vi "LinearBearingControl.vi"() -> ()   [LabVIEW 2012]
uses:
  stressTestTypeDef.ctl
  <vilib>/Utility/error.llb/DialogType.ctl
  allStatesTypeDef.ctl
  <vilib>/Analysis/baseanly.llb/Mean (DBL).vi
  <vilib>/Utility/file.llb/Write To Spreadsheet File (DBL).vi
  <resource>/objmgr/daqmx.rc
  <vilib>/Analysis/NI_AALBase.lvlib
panel:
  out "Force":dbl[](array[numeric]) format="%#.2g"
  out "Measurement":dbl[](graph)
  out "Bias (N)":dbl
  in  "Channel Parameters":T1={"Maximum Value"=10.0, "Minimum Value"=-10.0, "Channel"="Dev2/ai7"}
  in  "pulse/rev":u16(ring)=25600 items=["400"=400, "800"=800, "1600"=1600, "3200"=3200, "6400"=6400, "12800"=12800, "25600"=25600]
  out "concatenated string":string
  out "rigid body LED":bool
  out "strain rate":dbl
  in  "chain L0":i32=230
  out "mm/s (timed)":dbl
  in  "Direction":bool
  in  "Only Move Lin":bool
  out "writing data":bool
  out "stop sys":bool
  out "udp error out":errorcluster
  out "Voltages":dbl[](array[numeric])
  in  "Start System":bool
  in  "Auto Bias":bool=TRUE
  in  "Unbias":bool
  in  "Bias":bool
  in  "Collect Data":bool=TRUE
  in  "Timing parameters":T2={"Sample Rate"=1000.0, "Samples to Read"=100}
  out "filenameOut":string
  in  "Optitrack Parameters":T3={"Optitrack IP"="130.207.141.229", "Optitrack Port"=1520, "timeout (sec)"=80}
  out "Data Output File":path
  in  "Output Folder":path=path "C:/Users/Administrator/Dropbox/expData/chainData"
  in  "Program Parameters":T5={"v"=2500, "Iters"=2, "Speed"=5, "Delay"=0.5, "H"=11.5, "SD"=10, "Name"="Stretch", "Type"=enum."FRACT ON"} {"Speed" min=0 max=49 step=5}
  out "strain %":dbl
  out "FT error out":errorcluster
  # "for 6 smarts\nSDmax ~ 170mm"
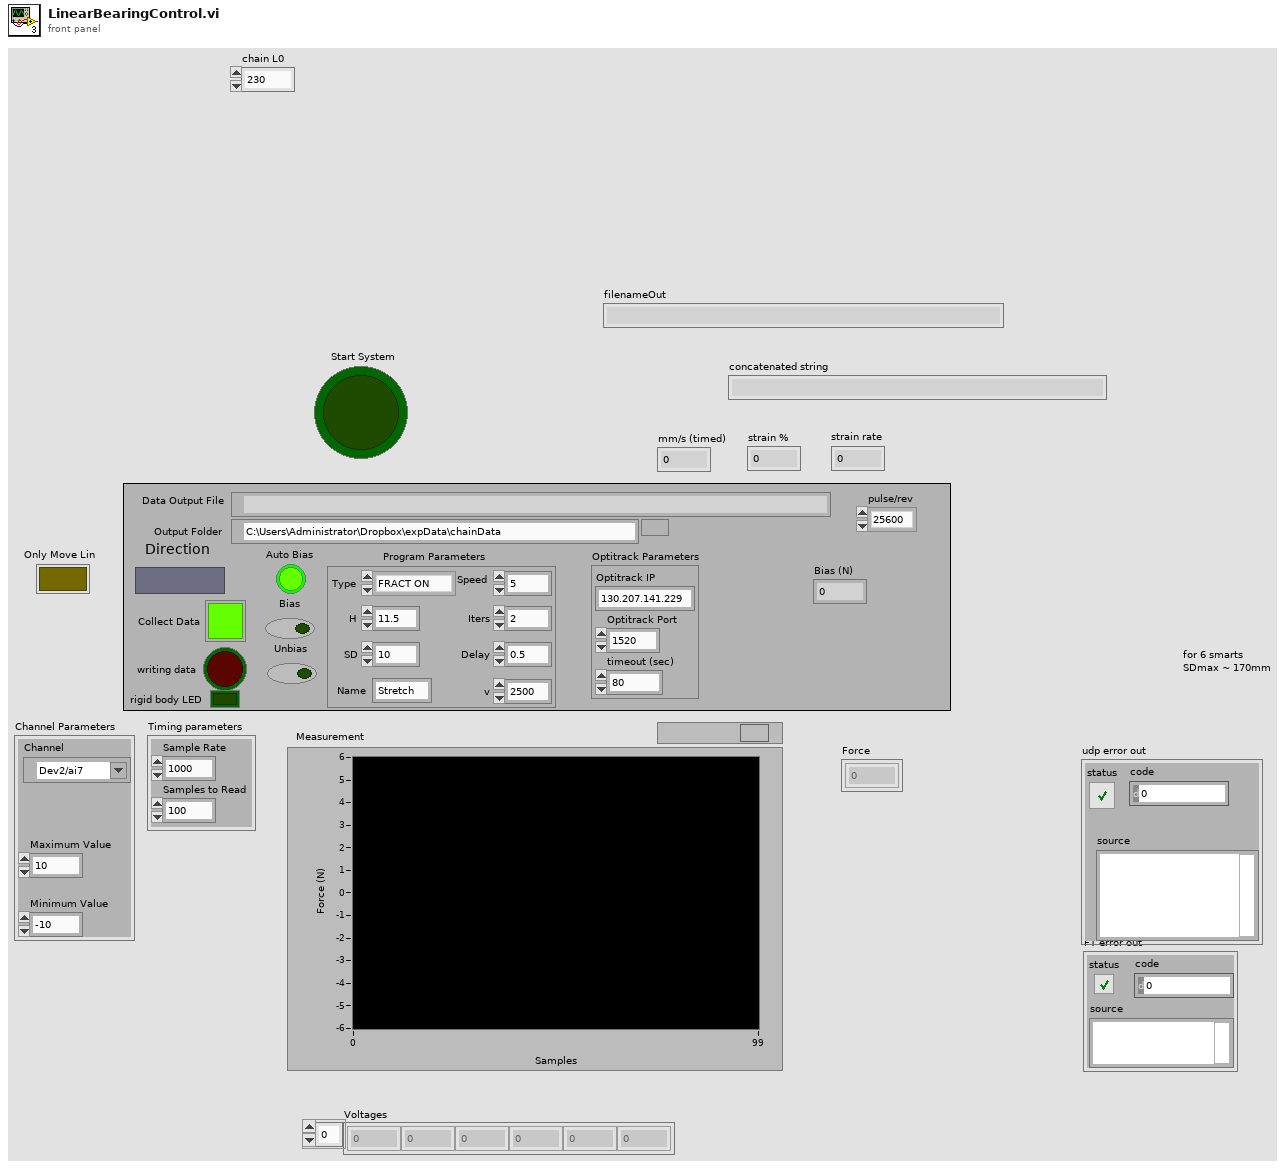
[diagram p1: front panel]
types:
  T1 = cluster{"Maximum Value":dbl, "Minimum Value":dbl, "Channel":tag}
  T2 = cluster{"Sample Rate":dbl, "Samples to Read":i32}
  T3 = cluster{"Optitrack IP":string, "Optitrack Port":u16, "timeout (sec)":i32}
  T4 = typedef "stressTestTypeDef.ctl" = enum16{"OFF", "ON", "EXTEND", "SPRING", "FRACT ON", "SAC", "FRACT SAC"}
  T5 = cluster{"v":i32, "Iters":i32, "Speed":i32, "Delay":dbl, "H":dbl, "SD":i32, "Name":string, "Type":T4}
  T6 = cluster{"distance mm":i32, "Direction":bool, "device name":tag, "speed (mm/s)":i32, "pulse/rev":u16}
  T7 = typedef "DialogType.ctl" = u16
  T8 = cluster{"SD":i32, "Delay":dbl, "Speed":i32, "Iters":i32, "Type":T4, "timeout":i32}
  T9 = typedef "allStatesTypeDef.ctl" = enum16{"open udp", "start record", "recording", "move linear actuator", "end record", "close udp", "end"}
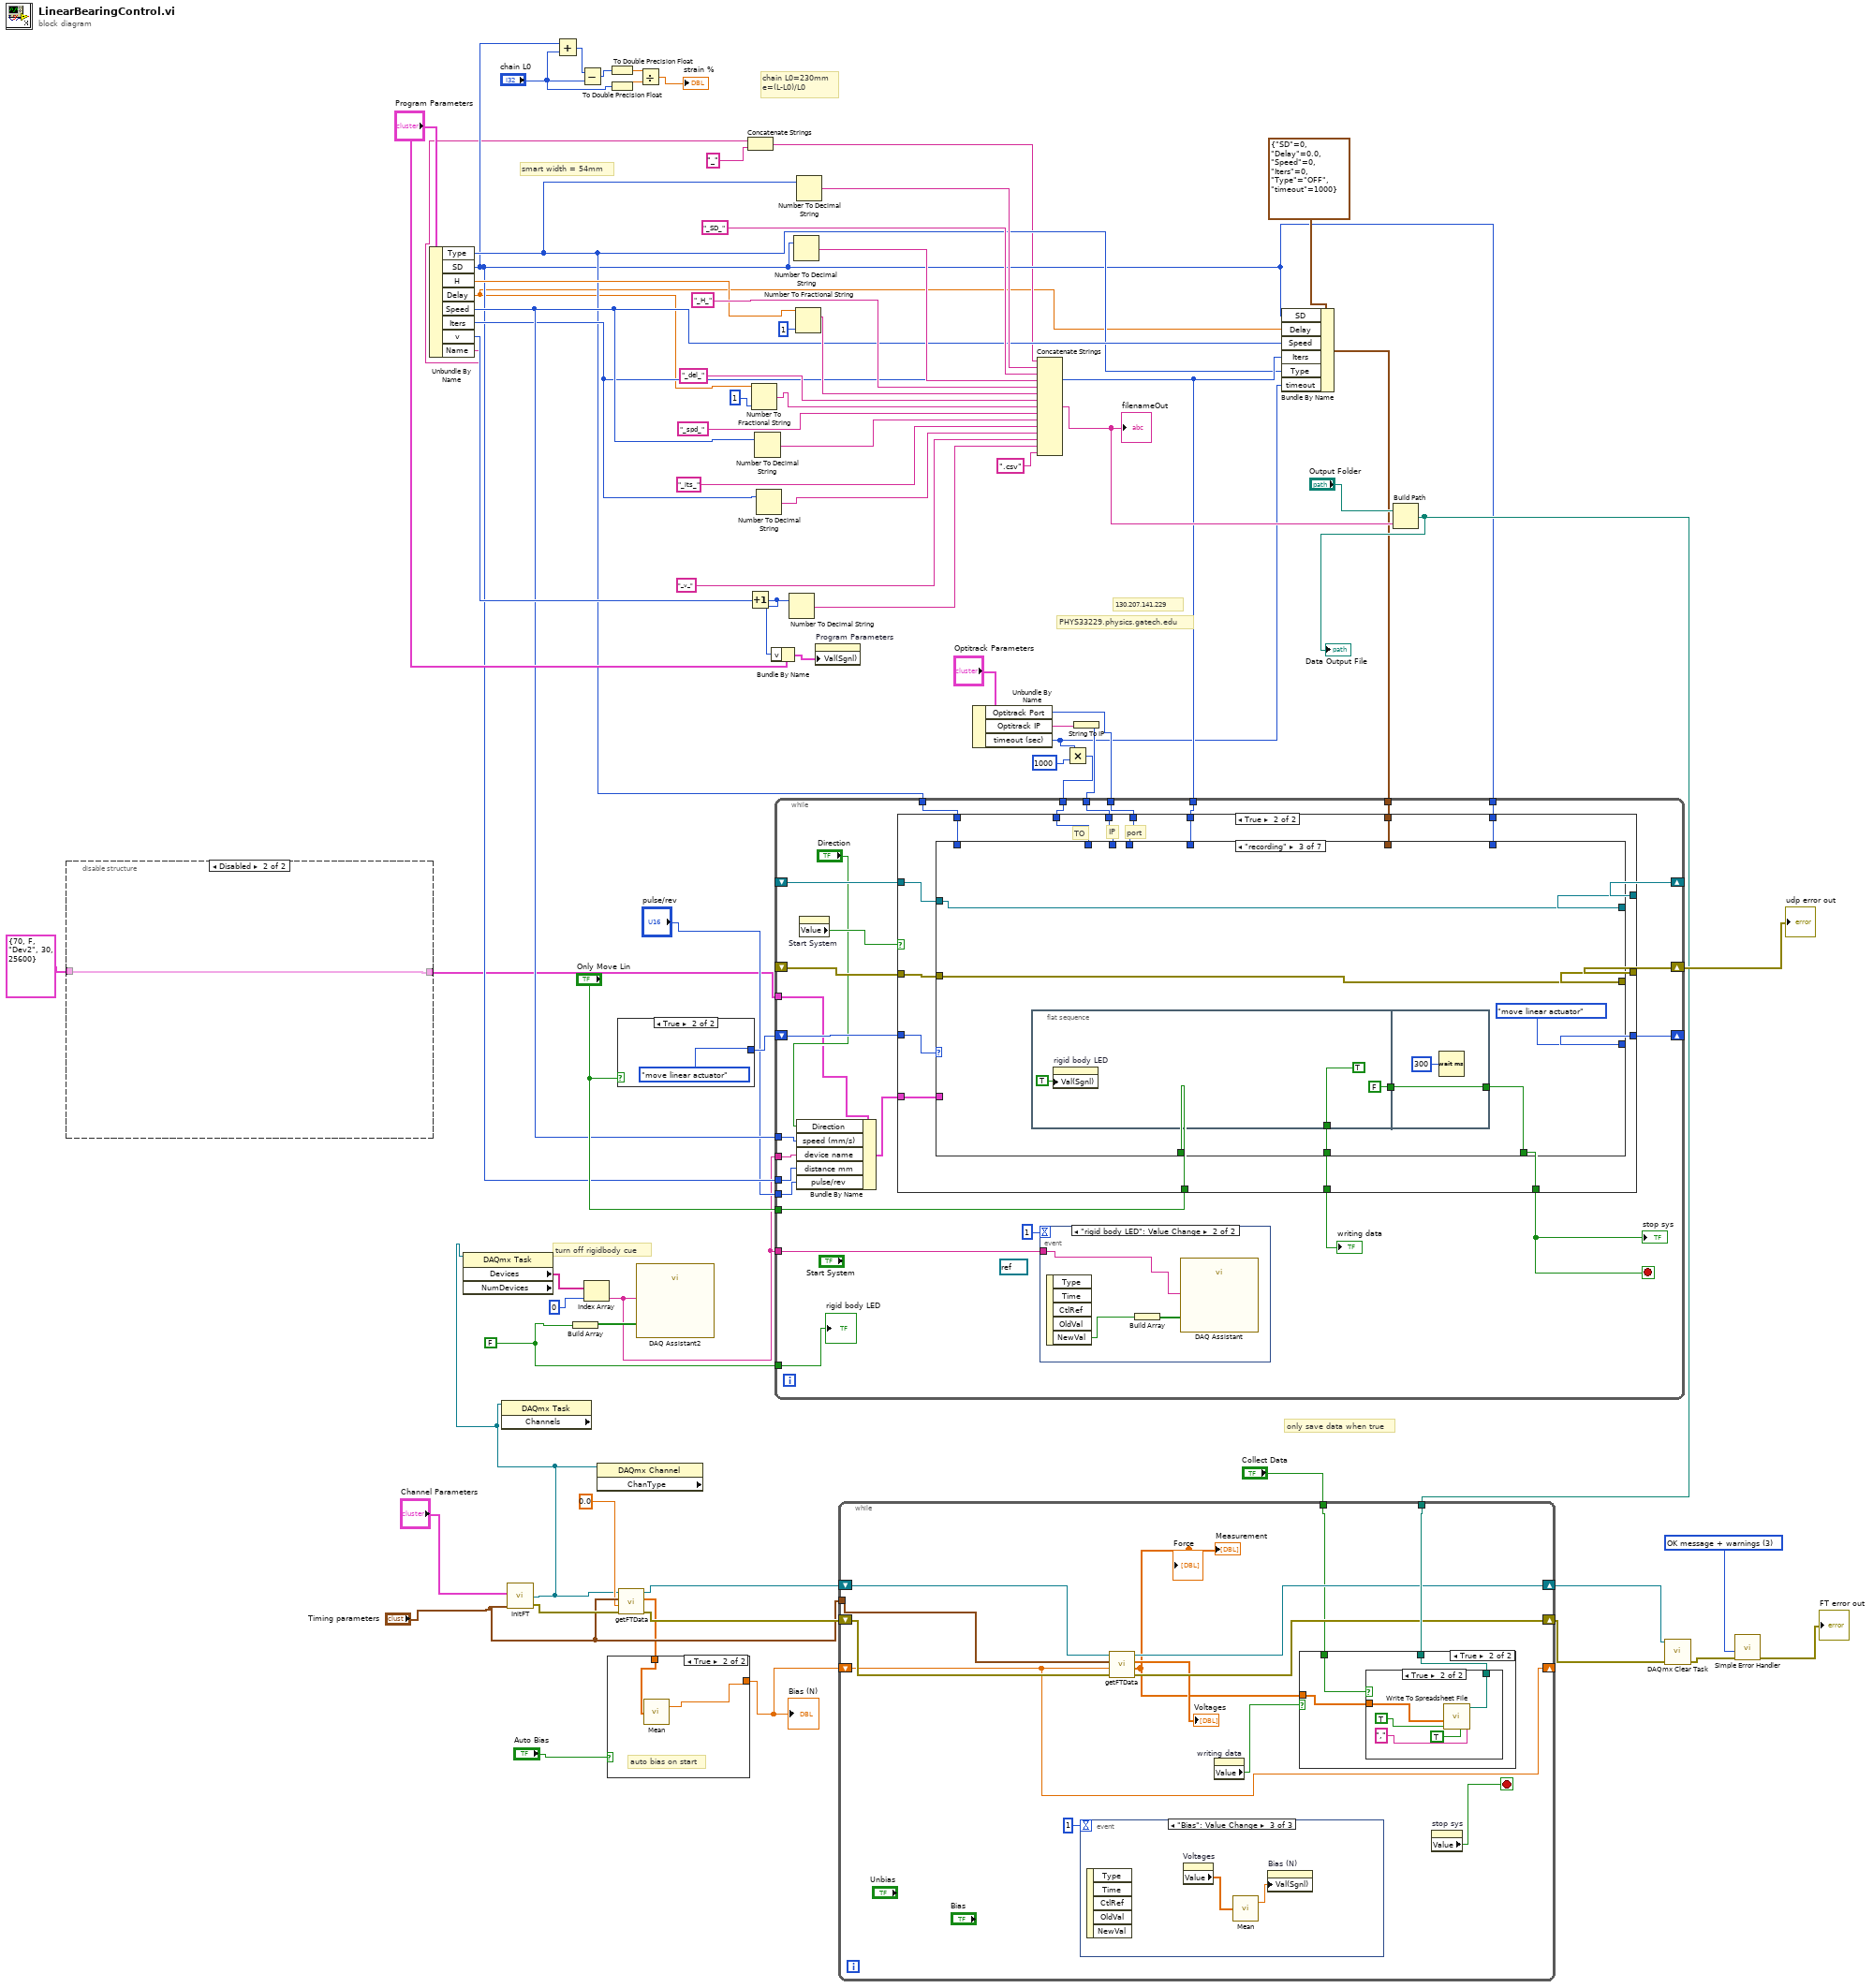
[diagram p0: block diagram]
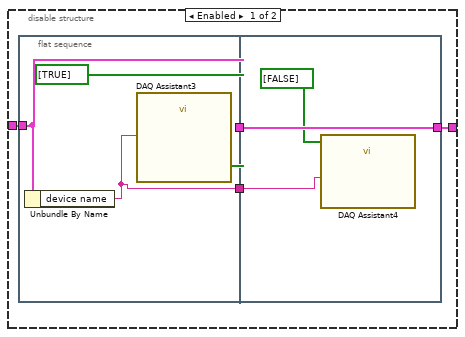
[diagram p2: hidden frame]
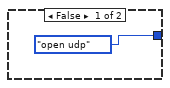
[diagram p3: hidden frame]
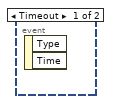
[diagram p4: hidden frame]
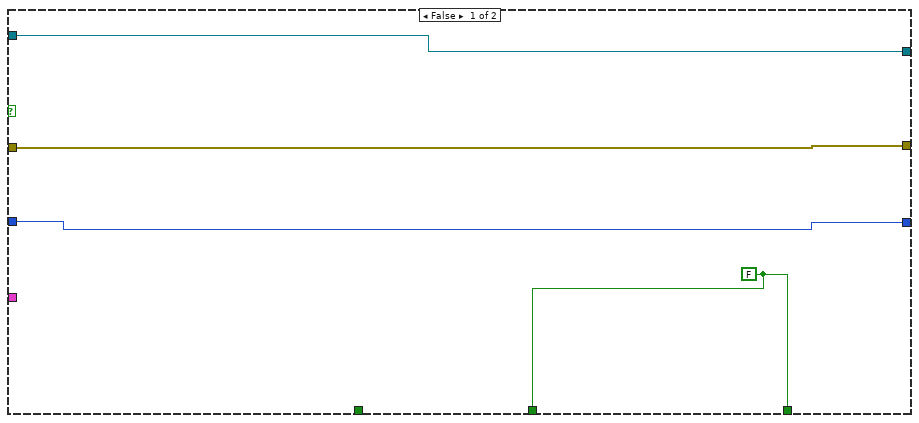
[diagram p5: hidden frame]
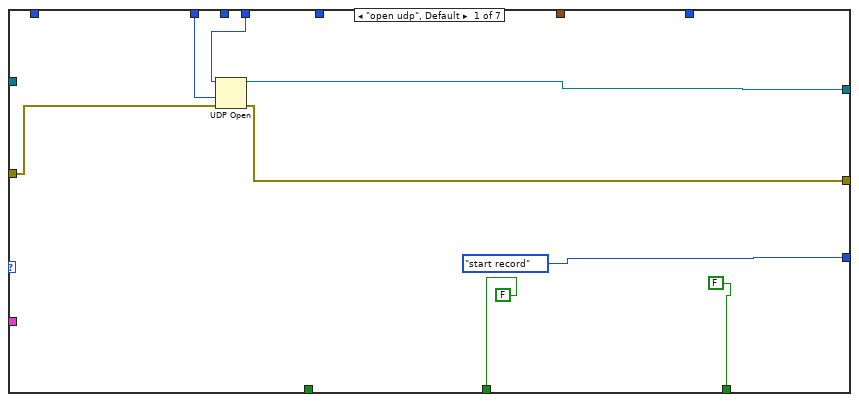
[diagram p6: hidden frame]
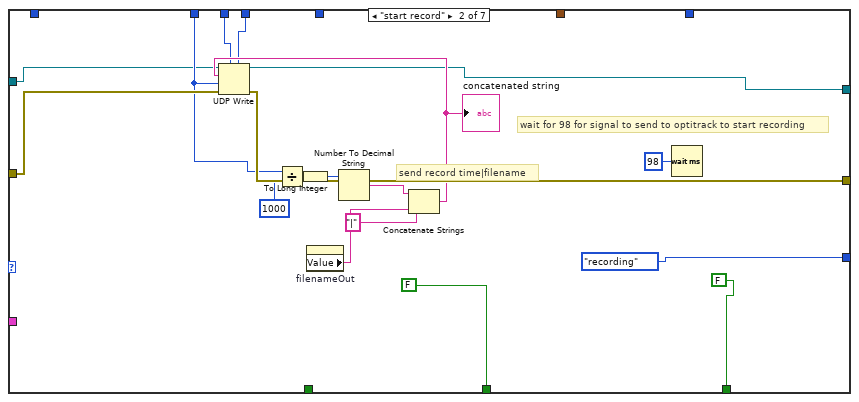
[diagram p7: hidden frame]
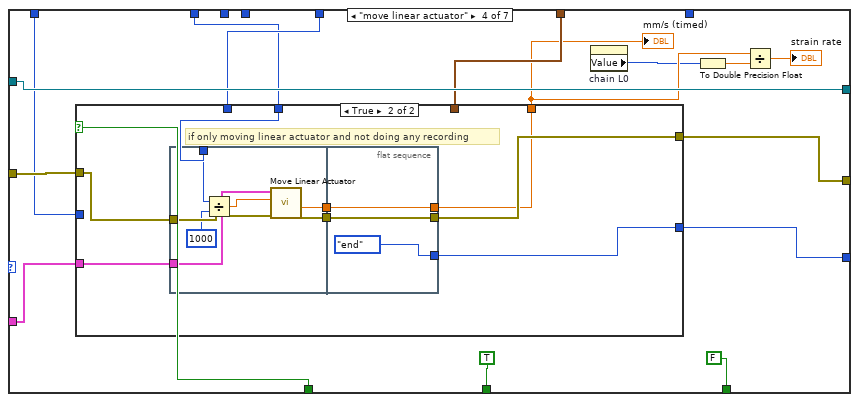
[diagram p8: hidden frame]
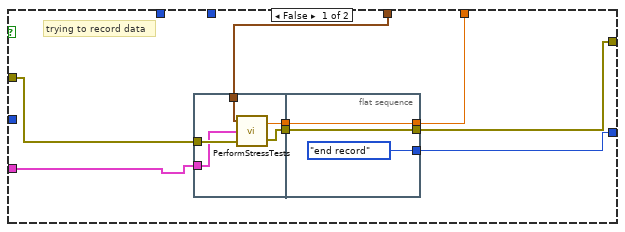
[diagram p9: hidden frame]
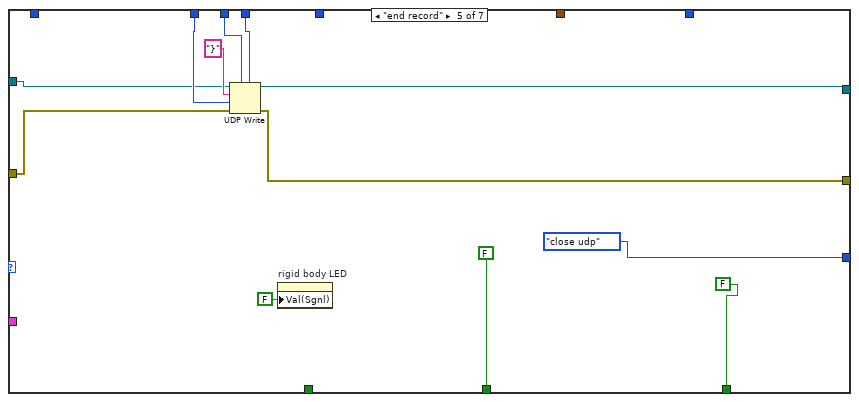
[diagram p10: hidden frame]
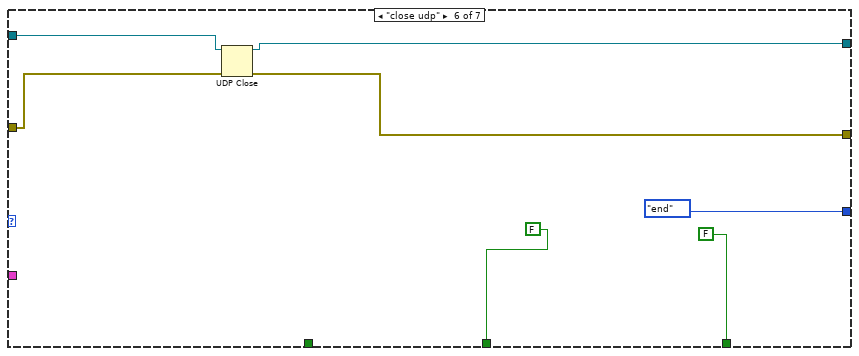
[diagram p11: hidden frame]
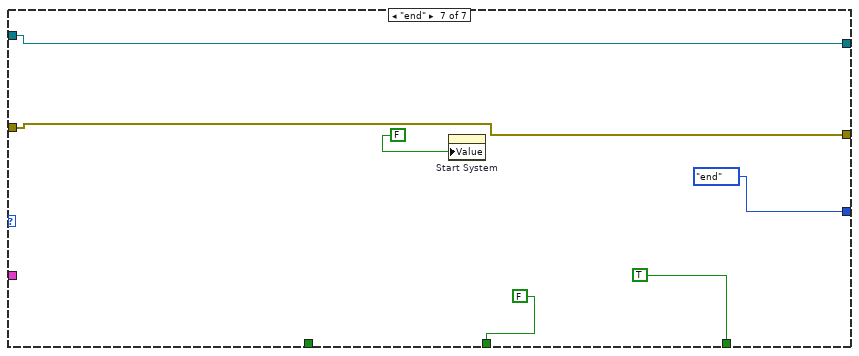
[diagram p12: hidden frame]
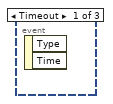
[diagram p13: hidden frame]
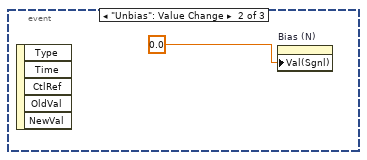
[diagram p14: hidden frame]
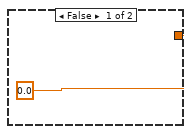
[diagram p17: hidden frame]
diagram:
  w19 = FALSE
  w47 = T7 3 items=["no dialog", "OK message", "continue or stop message", "OK message + warnings", "continue/stop + warnings"] ("type of dialog (OK msg:1)")
  # "turn off rigidbody cue"
  # "chain L0=230mm\ne=(L-L0)/L0"
  # "only save data when true"
  # "smart width = 54mm"
  # "PHYS33229.physics.gatech.edu"
  # "130.207.141.229"
  n1 = disable-structure shown="Disabled" {
    disable-tunnel: [w76 w85] -> w10
    disable-tunnel: T6 {"distance mm"=70, "Direction"=FALSE, "device name"="Dev2", "speed (mm/s)"=30, "pulse/rev"=25600} ("linear actuator info") -> [w75 w85]
    frame Enabled {
      n2 = flat-sequence {
        tunnel: w75 -> [w81]
        tunnel: [w81] -> w78
        tunnel: [w79] -> w77
        tunnel: [w84] -> w76
        tunnel: w78 -> [w84]
        tunnel: w77 -> [w83]
        frame #0 {
          n3 = Unbundle By Name(w81) -> ("device name"=w79:tag)
          n4 = call "DAQ Assistant3"("data"=bool[] [TRUE], "device name"=w79) -> ()  [unwired: 16 in, 2 out]
        }
        frame #1 {
          n5 = call "DAQ Assistant4"("data"=bool[] [FALSE], "device name"=w83) -> ()  [unwired: 16 in, 2 out]
        }
      }
    }
    frame Disabled {
    }
  }
  n6 = Unbundle By Name("Program Parameters") -> ("Type"=w29:T4, "SD"=w21:i32, "H"=w56:dbl, "Delay"=w13:dbl, "Speed"=w31:i32, "Iters"=w30:i32, "v"=w57:i32, "Name"=w16:string)
  n7 = call "InitFT.vi"("Timing parameters"="Timing parameters", "Channel Parameters"="Channel Parameters") -> ("error out"=w44:errorcluster, "task out"=w6:refnum<k21>)  [unwired: 3 in]
  n8 = property class="DAQmx Task" props=["Devices", "NumDevices"](reference=w6) -> ("Devices"=w3:tag[])  [unwired: 1 in, 3 out]
  n9 = property class="DAQmx Task" props=["Channels"](reference=w6) -> ()  [unwired: 1 in, 3 out]
  n10 = Add(x=w21, y="chain L0") -> (x+y=w27:i32)
  n11 = Build Array(w19) -> (w20:bool[])
  n12 = Subtract(x=w27, y="chain L0") -> (x-y=w26:i32)
  n13 = Index Array(array=w3, index=0) -> (element=w5:tag)
  n14 = property class="DAQmx Channel" props=["ChanType"](reference=w6) -> ()  [unwired: 1 in, 3 out]
  n15 = To Double Precision Float(number=w26) -> (double precision float=w24:dbl)
  n16 = To Double Precision Float(number="chain L0") -> (double precision float=w23:dbl)
  n17 = case shown="True" "Only Move Lin" {
    tunnel: [allStatesTypeDef."open udp" allStatesTypeDef."move linear actuator"] -> w74
    frame False {
    }
    frame True {
    }
  }
  n18 = call "getFTData.vi"("error in"=w44, "bias"=0.0, "Timing parameters"="Timing parameters", "task in"=w6) -> ("error out"=w40:errorcluster, "Voltage"=w2:dbl[], "task out 2"=w41:refnum<k21>)  [unwired: 1 in, 1 out]
  n19 = case shown="True" "Auto Bias" {
    tunnel: w2 -> [_ w90]
    tunnel: [0.0 ("Bias (N) 2") w89] -> w1
    frame False {
    }
    frame True {
      # "auto bias on start"
      n20 = call-poly <vilib>:"Mean.vi"("X"=w90) -> ("mean"=w89:dbl)  [unwired: 1 out]
    }
  }
  "Bias (N)" <- w1
  n21 = call "DAQ Assistant2"("data"=w20, "device name"=w5) -> ()  [unwired: 16 in, 2 out]
  n22 = Divide(x=w24, y=w23) -> (x/y=→"strain %":dbl)
  n23 = Concatenate Strings(w16, "_") -> (w17:string)
  n24 = Increment(x=w57) -> (x+1=w58:i32)
  n25 = Number To Fractional String(number=w13, precision (6)=i16 1) -> (F-format string=w11:string)  [unwired: 2 in]
  n26 = Number To Decimal String(number=w31) -> (decimal integer string=w62:string)  [unwired: 1 in]
  n27 = Number To Decimal String(number=w30) -> (decimal integer string=w60:string)  [unwired: 1 in]
  n28 = Bundle By Name(cluster="Program Parameters", "v"=w58) -> (w54:T5)
  n29 = Number To Decimal String(number=w58) -> (decimal integer string=w64:string)  [unwired: 1 in]
  n30 = Number To Decimal String(number=w21) -> (decimal integer string=w70:string)  [unwired: 1 in]
  n31 = Number To Fractional String(number=w56, precision (6)=i16 1) -> (F-format string=w67:string)  [unwired: 2 in]
  n32 = Number To Decimal String(number=w29) -> (decimal integer string=w72:string)  [unwired: 1 in]
  n33 = property on="Program Parameters" class="Clust (strict)"("Val(Sgnl)"=w54) -> ()  [unwired: 2 in, 2 out]
  n34 = Unbundle By Name("Optitrack Parameters") -> ("Optitrack Port"=w52:u16, "Optitrack IP"=w51:string, "timeout (sec)"=w15:i32)
  n35 = Concatenate Strings(w17, w72, "_SD_", w70, "_H_", w67, "_del_", w11, "_spd_", w62, "_its_", w60, "_v_", w64, ".csv") -> (w33:string)
  "filenameOut" <- w33
  n36 = Multiply(x=w15, y=1000) -> (x*y=w48:i32)
  n37 = String To IP(1:w51) -> (0:w50:u32)
  n38 = Bundle By Name(cluster=T8 {"SD"=0, "Delay"=0.0, "Speed"=0, "Iters"=0, "Type"=enum."OFF", "timeout"=1000}, "SD"=w21, "Delay"=w13, "Speed"=w31, "Iters"=w30, "Type"=w29, "timeout"=w15) -> (w28:T8)
  n39 = while {
    shift-right: [w117] -> w36
    shift-left: _ -> [w116]
    shift-right: [w114] -> _
    shift-left: w74 -> [w115]
    tunnel: w52 -> [w112]
    tunnel: w50 -> [w113]
    tunnel: w48 -> [w93]
    shift-right: [w111] -> _
    shift-left: _ -> [w110]
    tunnel: "Only Move Lin" -> [w107]
    tunnel: w31 -> [w104]
    tunnel: w21 -> [w95]
    tunnel: w29 -> [w103]
    tunnel: w30 -> [w102]
    tunnel: w28 -> [w101]
    tunnel: w21 -> [w99]
    tunnel: w19 -> [w98]
    tunnel: w5 -> [w96]
    tunnel: w5 -> [w94]
    tunnel: "pulse/rev" -> [w92]
    tunnel: w10 -> [w91]
    stop <- w109 stop-if-true
    (unwired) refnum<k21> refnum ("Name")
    n40 = Bundle By Name(cluster=w91, "Direction"="Direction", "speed (mm/s)"=w104, "device name"=w96, "distance mm"=w95, "pulse/rev"=w92) -> (w106:T6)
    n41 = property on="Start System" class="Bool (strict)"() -> ("Value"=w108:bool)  [unwired: 2 in, 2 out]
    n42 = case shown="True" w108 {
      tunnel: [w121 w141] -> w117
      tunnel: w116 -> [w121 w140]
      tunnel: w115 -> [w124 w139]
      tunnel: [w124 w138] -> w114
      tunnel: w113 -> [_ w137]
      tunnel: w112 -> [_ w130]
      tunnel: w93 -> [_ w136]
      tunnel: [w122 w135] -> w111
      tunnel: w110 -> [w122 w134]
      tunnel: [w123 w133] -> w100
      tunnel: [w123 w132] -> w109
      tunnel: w107 -> [_ w131]
      tunnel: w106 -> [_ w129]
      tunnel: w103 -> [_ w128]
      tunnel: w102 -> [_ w127]
      tunnel: w101 -> [_ w126]
      tunnel: w99 -> [_ w125]
      frame False {
        w123 = FALSE
      }
      frame True {
        # "IP"
        # "TO"
        # "port"
        n43 = case shown="\"recording\"" w139 {
          tunnel: w136 -> [w146 w159 _ w179 w236 _ _]
          tunnel: w140 -> [w147 w165 w169 w190 w240 w246 w248]
          tunnel: [w148 w166 w169 w189 w239 w247 w248] -> w141
          tunnel: [allStatesTypeDef."start record" allStatesTypeDef."recording" allStatesTypeDef."move linear actuator" w192 allStatesTypeDef."close udp" allStatesTypeDef."end" allStatesTypeDef."end"] -> w138
          tunnel: [FALSE FALSE w171 FALSE FALSE FALSE TRUE] -> w132
          tunnel: w137 -> [_ w152 _ _ w230 _ _]
          tunnel: [w145 w155 w170 w191 w234 w245 w253] -> w135
          tunnel: w134 -> [_ w156 w170 w191 w233 w241 w253]
          tunnel: [FALSE FALSE w172 TRUE FALSE FALSE FALSE] -> w133
          tunnel: w131 -> [_ _ _ w188 _ _ _]
          tunnel: w130 -> [w142 w151 _ _ w231 _ _]
          tunnel: w129 -> [_ _ _ w187 _ _ _]
          tunnel: w128 -> [_ _ _ w185 _ _ _]
          tunnel: w127 -> [_ _ _ w186 _ _ _]
          tunnel: w126 -> [_ _ _ w184 _ _ _]
          tunnel: w125 -> [_ _ _ _ _ _ _]
          frame "open udp", Default {
            n44 = UDP Open(8:w147, 9:w146, 11:w142) -> (port=w145:refnum<k16>, 0:w148:errorcluster)  [unwired: 2 in, 1 out]
          }
          frame "start record" {
            # "wait for 98 for signal to send to optitrack to start recording"
            # "send record time|filename"
            n45 = Divide(x=w159, y=1000) -> (x/y=w158:dbl)
            n46 = To Long Integer(number=w158) -> (32bit integer=w157:i32)
            n47 = property on="filenameOut" class="Str"() -> ("Value"=w163:string)  [unwired: 2 in, 2 out]
            n48 = Number To Decimal String(number=w157) -> (decimal integer string=w161:string)  [unwired: 1 in]
            n49 = Concatenate Strings(w161, "|" ("string"), w163) -> (w162:string)
            "concatenated string" <- w162
            n50 = UDP Write(address=w152, port or service name=w151, connection ID=w156, data in=w162, 8:w165, 9:w159) -> (error out=w166:errorcluster, 3:w155:refnum<k16>)
            n51 = Wait (ms)(milliseconds to wait=u32 98) -> ()  [unwired: 1 out]
          }
          frame "recording" {
            n52 = flat-sequence {
              tunnel: [TRUE] -> w172
              tunnel: [FALSE] -> w168
              tunnel: [w178] -> w171
              tunnel: w168 -> [w178]
              frame #0 {
                n53 = property on="rigid body LED" class="Bool (strict)"("Val(Sgnl)"=TRUE ("Value (Signaling)")) -> ()  [unwired: 2 in, 2 out]
              }
              frame #1 {
                n54 = Wait (ms)(milliseconds to wait=u32 300) -> ()  [unwired: 1 out]
              }
            }
          }
          frame "move linear actuator" {
            n55 = case shown="True" w188 {
              tunnel: [w195 w212] -> w192
              tunnel: w190 -> [w199 w216]
              tunnel: [w198 w217] -> w189
              tunnel: w187 -> [w200 w218]
              tunnel: [w201 w215] -> w183
              tunnel: w186 -> [_ _]
              tunnel: w185 -> [_ _]
              tunnel: w184 -> [w202 _]
              tunnel: w179 -> [_ w211]
              frame False {
                # "trying to record data"
                n56 = flat-sequence {
                  tunnel: w202 -> [w207]
                  tunnel: w200 -> [w203]
                  tunnel: w199 -> [w205]
                  tunnel: [w206] -> w197
                  tunnel: [w204] -> w196
                  tunnel: w197 -> [w210]
                  tunnel: w196 -> [w209]
                  tunnel: [w210] -> w201
                  tunnel: [w209] -> w198
                  tunnel: [allStatesTypeDef."end record"] -> w195
                  frame #0 {
                    n57 = call "PerformStressTests.vi"("error in"=w205, "linear actuator info"=w203, "Test Info"=w207) -> ("error out"=w204:errorcluster, "mm/s (timed)"=w206:dbl)
                  }
                  frame #1 {
                  }
                }
              }
              frame True {
                # "if only moving linear actuator and not doing any recording"
                n58 = flat-sequence {
                  tunnel: w218 -> [w225]
                  tunnel: w216 -> [w223]
                  tunnel: [w224] -> w214
                  tunnel: [w222] -> w213
                  tunnel: w211 -> [w220]
                  tunnel: w214 -> [w228]
                  tunnel: w213 -> [w227]
                  tunnel: [w228] -> w217
                  tunnel: [w227] -> w215
                  tunnel: [allStatesTypeDef."end"] -> w212
                  frame #0 {
                    n59 = Divide(x=w220, y=1000) -> (x/y=w219:dbl)
                    n60 = call "Move Linear Actuator.vi"("error in"=w223, "timeout"=w219, "linear actuator info"=w225) -> ("error out"=w224:errorcluster, "mm/s (timed)"=w222:dbl)  [unwired: 1 in, 1 out]
                  }
                  frame #1 {
                  }
                }
              }
            }
            "mm/s (timed)" <- w183
            n61 = property on="chain L0" class="DigNum (strict)"() -> ("Value"=w182:i32)  [unwired: 2 in, 2 out]
            n62 = To Double Precision Float(number=w182) -> (double precision float=w181:dbl)
            n63 = Divide(x=w183, y=w181) -> (x/y=→"strain rate":dbl)
          }
          frame "end record" {
            n64 = UDP Write(address=w230, port or service name=w231, connection ID=w233, data in="}", 8:w240, 9:w236) -> (error out=w239:errorcluster, 3:w234:refnum<k16>)
            n65 = property on="rigid body LED" class="Bool (strict)"("Val(Sgnl)"=FALSE ("Value (Signaling)")) -> ()  [unwired: 2 in, 2 out]
          }
          frame "close udp" {
            n66 = UDP Close(connection ID=w241, 8:w246) -> (connection ID out=w245:refnum<k16>, error out=w247:errorcluster)
          }
          frame "end" {
            n67 = property on="Start System" class="Bool (strict)"("Value"=FALSE) -> ()  [unwired: 2 in, 2 out]
          }
        }
      }
    }
    "stop sys" <- w109
    "writing data" <- w100
    n68 = event shown="[1] \"rigid body LED\": Value Change" {
      selector: _ -> [_ _]
      dyn-events: _ -> [_ _]
      timeout: 1 -> [_ _]
      tunnel: w94 -> [_ w118]
      event Timeout {
        n69 = event-data() -> ()  [unwired: 1 in, 2 out]
      }
      event "rigid body LED": Value Change {
        n70 = event-data() -> ("NewVal"=w119:bool)  [unwired: 1 in, 4 out]
        n71 = Build Array(w119) -> (w120:bool[])
        n72 = call "DAQ Assistant"("data"=w120, "device name"=w118) -> ()  [unwired: 16 in, 2 out]
      }
    }
    "rigid body LED" <- w98
  }
  "udp error out" <- w36
  n73 = Build Path(base path="Output Folder", name or relative path=w33) -> (appended path=w35:path)
  "Data Output File" <- w35
  n74 = while {
    tunnel: w35 -> [w266]
    tunnel: "Collect Data" -> [w258]
    shift-right: [w265] -> w38
    shift-left: w41 -> [w263]
    shift-right: [w261] -> w37
    shift-left: w40 -> [w264]
    tunnel: "Timing parameters" -> [w262]
    shift-right: [w254] -> _
    shift-left: w1 -> [w254]
    stop <- w259 stop-if-true
    n75 = event shown="[2] \"Bias\": Value Change" {
      selector: _ -> [_ _ _]
      dyn-events: _ -> [_ _ _]
      timeout: 1 -> [_ _ _]
      event Timeout {
        n76 = event-data() -> ()  [unwired: 1 in, 2 out]
      }
      event "Unbias": Value Change {
        n77 = event-data() -> ()  [unwired: 1 in, 5 out]
        n78 = property on="Bias (N)" class="DigNum (strict)"("Val(Sgnl)"=0.0 ("Bias (N) 2")) -> ()  [unwired: 2 in, 2 out]
      }
      event "Bias": Value Change {
        n79 = event-data() -> ()  [unwired: 1 in, 5 out]
        n80 = property on="Voltages" class="Arr (strict)"() -> ("Value"=w269:dbl[])  [unwired: 2 in, 2 out]
        n81 = call-poly <vilib>:"Mean.vi"("X"=w269) -> ("mean"=w268:dbl)  [unwired: 1 out]
        n82 = property on="Bias (N)" class="DigNum (strict)"("Val(Sgnl)"=w268) -> ()  [unwired: 2 in, 2 out]
      }
    }
    n83 = call "getFTData.vi"("error in"=w264, "bias"=w254, "Timing parameters"=w262, "task in"=w263) -> ("error out"=w261:errorcluster, "Force"=w255:dbl[], "Voltage"=→"Voltages":dbl[], "task out 2"=w265:refnum<k21>)  [unwired: 1 in]
    "Measurement" <- w255
    "Force" <- w255
    n84 = property on="writing data" class="Bool (strict)"() -> ("Value"=w257:bool)  [unwired: 2 in, 2 out]
    n85 = case shown="True" w257 {
      tunnel: w255 -> [_ w272]
      tunnel: w266 -> [_ w271]
      tunnel: w258 -> [_ w270]
      frame False {
      }
      frame True {
        n86 = case shown="True" w270 {
          tunnel: w272 -> [_ w274]
          tunnel: w271 -> [_ w277]
          frame False {
          }
          frame True {
            n87 = call-poly <vilib>:"Write To Spreadsheet File.vi"("delimiter (\\t)"=",", "transpose? (no:F)"=TRUE, "append to file? (new file:F)"=TRUE, "1D data"=w274, "file path (dialog if empty)"=w277) -> ()  [unwired: 3 in, 1 out]
          }
        }
      }
    }
    n88 = property on="stop sys" class="Bool (strict)"() -> ("Value"=w259:bool)  [unwired: 2 in, 2 out]
  }
  n89 = call <vilib>:"DAQmx Clear Task.vi"("task in"=w38, "error in"=w37) -> ("error out"=w45:errorcluster)  [unwired: 13 in]
  n90 = call <vilib>:"Simple Error Handler.vi"("type of dialog (OK msg:1)"=w47, "error in (no error)"=w45) -> ("error out"=→"FT error out":errorcluster)  [unwired: 3 in, 4 out]
